vi "Manage Collision.vi"(11 "Missile-Goal Post in":refnum<class "Missile-Goal Post.lvclass">) -> (1 "Remove GB Components out":refnum<class "Game Board Component.lvclass">[](array[class]), 2 "GB Components out":refnum<class "Game Board Component.lvclass">[](array[class]))   [LabVIEW 2021, in "Missile-Goal Post.lvclass"]
doc: "MIT Licence\nCopyright (c) 2024 David Grollier"
uses:
  Missile-Goal Post.lvclass
  C:/Users/David/Documents/GameSoccerSpace/Source/Collision/Collision.lvclass
  Game Componants/Game Board Component/Game Board Component.lvclass
  Game Componants/Game Board Component/Movable/Movable.lvclass
  C:/Users/David/Documents/GameSoccerSpace/Source/Game Componants/Game Board Component/Game Board Component.lvclass
  Collision.lvclass
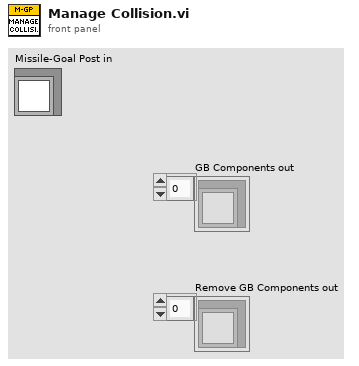
[diagram p1: front panel]
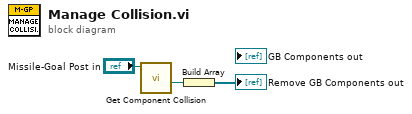
[diagram p0: block diagram]
diagram:
  n1 = call "Get Component Collision.vi"("Collision in"="Missile-Goal Post in") -> ("Movable out"=w3:refnum<class "Movable.lvclass">)  [unwired: 9 in, 1 out]
  n2 = Build Array(w3) -> (→"Remove GB Components out":refnum<class "Movable.lvclass">[])
